vi "Read program file.vi"(8 "error in (no error)":errorcluster, 11 "selected path":path) -> (0 "error out":errorcluster, 2 "text":string, 3 "Program out 2":T1[](array[typedef]))   [LabVIEW 2014]
uses:
  Teszt.ctl
  Command.ctl
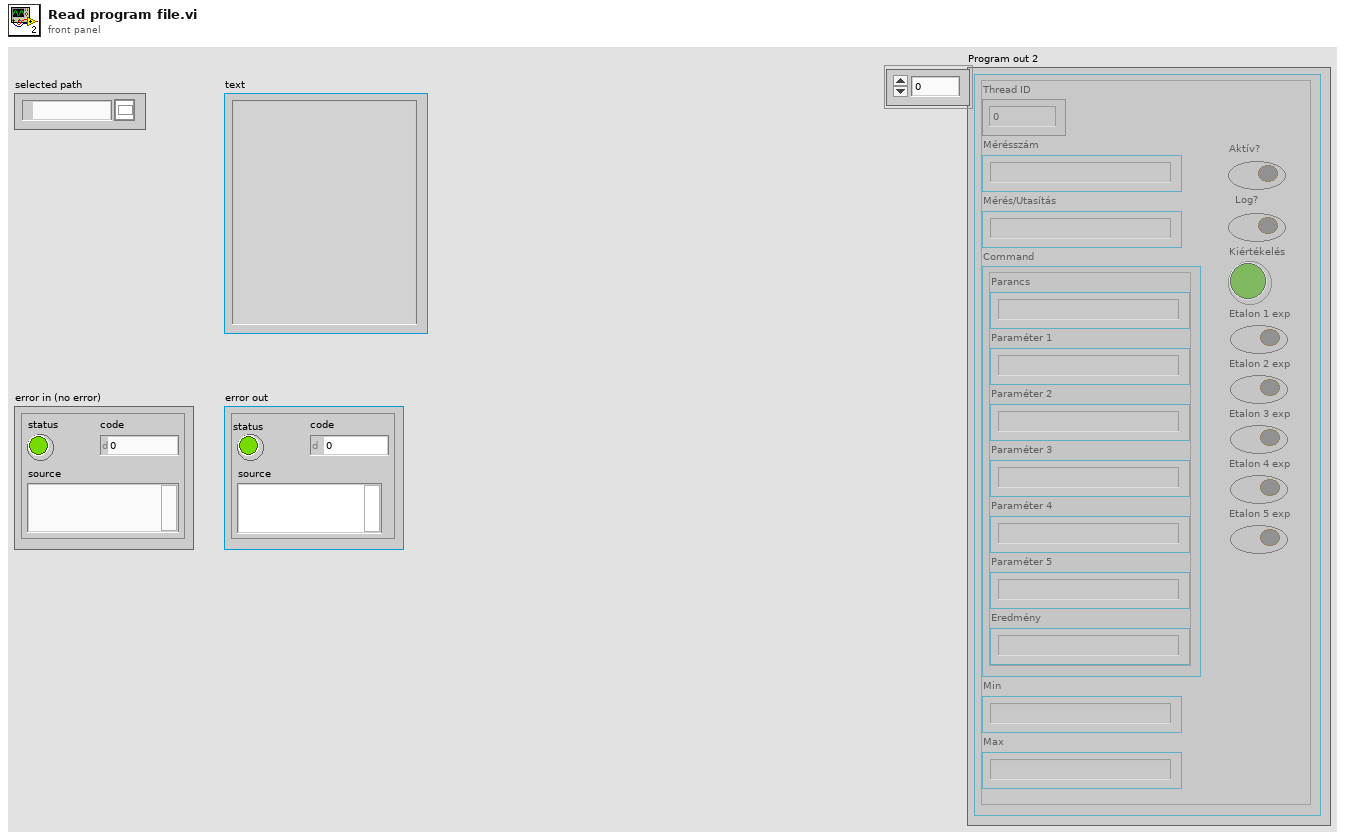
[diagram p1: front panel]
types:
  T1 = typedef "Teszt.ctl" = cluster{"Thread ID":dbl, "Mérésszám":string, "Mérés/Utasítás":string, "Command":T2, "Min":string, "Max":string, "Aktív?":bool, "Log?":bool, "Kiértékelés":bool, "Etalon 1 exp":bool, "Etalon 2 exp":bool, "Etalon 3 exp":bool, "Etalon 4 exp":bool, "Etalon 5 exp":bool}
  T2 = typedef "Command.ctl" = cluster{"Parancs":string, "Paraméter 1":string, "Paraméter 2":string, "Paraméter 3":string, "Paraméter 4":string, "Paraméter 5":string, "Eredmény":string}
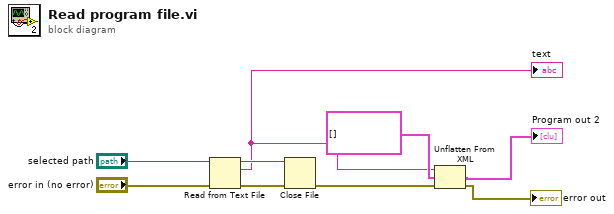
[diagram p0: block diagram]
diagram:
  n1 = Read from Text File(file (use dialog)="selected path", error in="error in (no error)") -> (refnum out=w5:refnum<file>, text=w2:string, error out=w4:errorcluster)  [unwired: 2 in, 1 out]
  "text" <- w2
  n2 = Close File(refnum=w5, error in=w4) -> (error out=w3:errorcluster)  [unwired: 1 out]
  n3 = Unflatten From XML(xml string=w2, type=T1[] [], error in (no error)=w3) -> (value=→"Program out 2":T1[], error out=→"error out":errorcluster)
